vi "Process Mouse Move.vi"(0 "State":T1={"Nspeakers"=13, "actions"=[], "Wspeaker"=13, "hover"={"type"=enum."None", "index"=0}, "locked"=FALSE, "states"=[], "sel speak"=13, "selected"=refnum, "Events"={"Selection change"=refnum}}, 5 "Layout":T6, 7 "Coords":T8) -> (8 "Hover Data":T2)   [LabVIEW 2015, in "SAC Config.xctl"]
uses:
  SAC Config.xctl
  <vilib>/Utility/miscctls.llb/LVPoint32TypeDef.ctl
  Layout.ctl
  Item.ctl
  Hover Data.ctl
  Hover Item.ctl
  State.vi
  Speaker State.ctl
  Events.ctl
  Selection changed.ctl
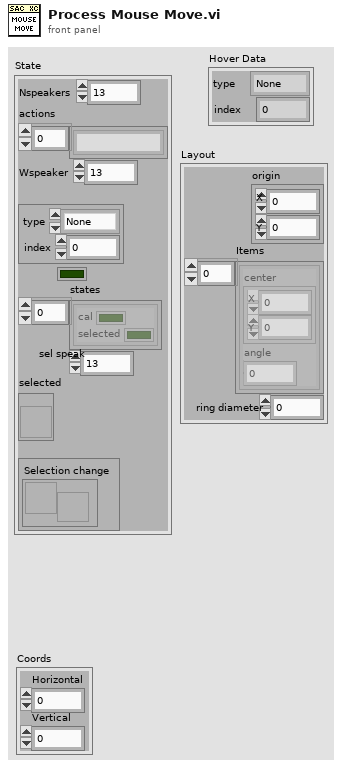
[diagram p1: front panel]
types:
  T1 = typedef "SAC Config.xctl/State.vi" = cluster{"Nspeakers":i32, "actions":string[], "Wspeaker":i32, "hover":T2, "locked":bool, "states":T4[], "sel speak":i32, "selected":refnum<vi>, "Events":T5}
  T2 = typedef "SAC Config.xctl/Hover Data.ctl" = cluster{"type":T3, "index":i32}
  T3 = typedef "SAC Config.xctl/Hover Item.ctl" = enum16{"None", "Speaker"}
  T4 = typedef "SAC Config.xctl/Speaker State.ctl" = cluster{"cal":bool, "selected":bool}
  T5 = typedef "SAC Config.xctl/Events.ctl" = cluster{"Selection change":refnum<user-event>}
  T6 = typedef "SAC Config.xctl/Layout.ctl" = cluster{"origin":cluster{"X":i32, "Y":i32}, "Items":T7[], "ring diameter":i32}
  T7 = typedef "SAC Config.xctl/Item.ctl" = cluster{"center":cluster{"X":i32, "Y":i32}, "angle":dbl}
  T8 = typedef "LVPoint32TypeDef.ctl" = cluster{"Horizontal":i32, "Vertical":i32}
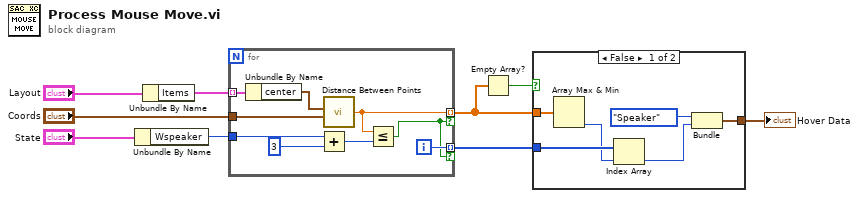
[diagram p0: block diagram]
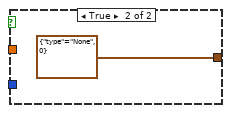
[diagram p2: hidden frame]
diagram:
  n1 = Unbundle By Name("State") -> ("Wspeaker"=w4:i32)
  n2 = Unbundle By Name("Layout") -> ("Items"=w7:T7[])
  n3 = for {
    tunnel: w7 -> [w18] mode=indexing
    tunnel: "Coords" -> [w17]
    tunnel: w4 -> [w16]
    tunnel: [w15] -> w1 mode=indexing if=w10
    tunnel: [w11] -> w2 mode=indexing if=w10
    i -> [w15]
    n4 = Unbundle By Name(w18) -> ("center"=w12:cluster{"X":i32, "Y":i32})
    n5 = Add(x=w16, y=3) -> (x+y=w14:i32)
    n6 = call "Distance Between Points.vi"("B"=w17, "A"=w12) -> ("distance"=w11:dbl)  [unwired: 4 in]
    n7 = Less Or Equal?(x=w11, y=w14) -> (x <= y?=w10:bool)
  }
  n8 = Empty Array?(array=w2) -> (empty?=w3:bool)
  n9 = case shown="False" w3 {
    tunnel: [w23 cluster{"type":T3, i32} {"type"=enum."None", 0}] -> w9
    tunnel: w2 -> [w22 _]
    tunnel: w1 -> [w21 _]
    frame False {
      n10 = Array Max & Min(array=w22) -> (min index (indices)=w20:i32)  [unwired: 3 out]
      n11 = Index Array(array=w21, index=w20) -> (element=w19:i32)
      n12 = Bundle("type"=Hover_Item."Speaker", w19) -> (w23:cluster{"type":T3, i32})  [unwired: 1 in]
    }
    frame True {
    }
  }
  "Hover Data" <- w9
